vi "Set Error Color.vi"(8 "error in (no error)":errorcluster caption="错误输入（无错误）", 10 "Error Color":u32(colorbox), 11 "SpecificString 输入":refnum<class "SpecificString.lvclass">) -> (0 "error out":errorcluster caption="错误输出", 3 "SpecificString 输出":refnum<class "SpecificString.lvclass">)   [LabVIEW 2018, in "SpecificString.lvclass"]
uses:
  SpecificString.lvclass
  SpecificString.lvclass/SpecificString.ctl
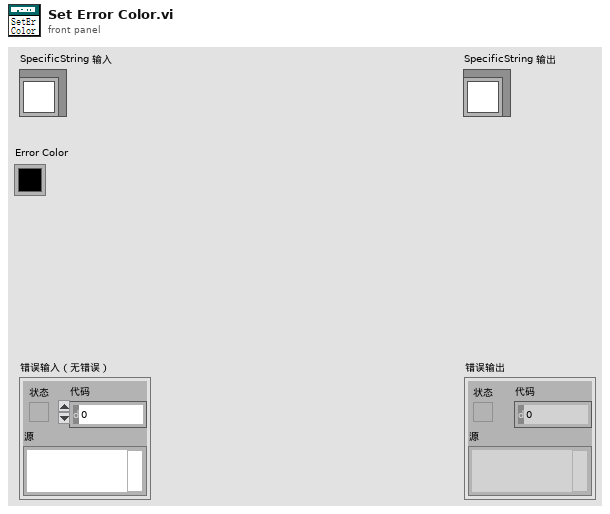
[diagram p1: front panel]
types:
  T1 = typedef "SpecificString.lvclass/State Data.ctl" = cluster{"Format":string, "Correct Color":u32, "Error Color":u32}
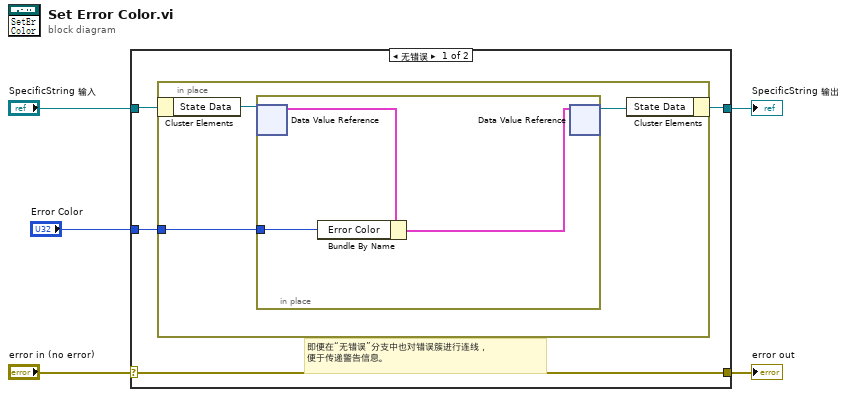
[diagram p0: block diagram]
diagram:
  n1 = case shown="无错误" "error in (no error)" {
    selector: "error in (no error)" -> [w9 w17]
    tunnel: [w9 w17] -> w4
    tunnel: [w7 w16] -> w2
    tunnel: "SpecificString 输入" -> [w8 w16]
    tunnel: "Error Color" -> [w6 _]
    frame No Error {
      # "即便在“无错误”分支中也对错误簇进行连线，\n便于传递警告信息。"
      n2 = in-place {
        in-place-border: w6 -> [w10]
        n3 = in-place-cluster #1(w8) -> ("State Data"=w12:refnum<data-value>)
        n4 = in-place {
          in-place-border: w10 -> [w13]
          n5 = in-place-dvr #2(w12) -> (w15:T1)  [unwired: 1 out]
          n6 = Bundle By Name(cluster=w15, "Error Color"=w13) -> (w14:T1)
          n7 = in-place-dvr #2(w14) -> (w11:refnum<data-value>)  [unwired: 1 out]
        }
        n8 = in-place-cluster #1("State Data"=w11) -> (w7:refnum<class "SpecificString.lvclass">)
      }
    }
    frame Error {
    }
  }
  "error out" <- w4
  "SpecificString 输出" <- w2
